vi "Eurotherm 32xx Series Temperature Control Monitoring.vi"() -> ()   [LabVIEW 2010]
doc: "This example demonstrates temperature control and monitoring.\n\nNote:\nBefore start this VI is it necessary:\n\n- preconfigure some specific parameters that are not supported by this driver (e.g. PV-I/O Type, Linearization type, Alarm Input Values... ) by Quick Codes, or by Eurotherm iTools or by instrument front panel controls\n- enter correct VISA Resource Descriptor, Device Address and Baud Rate into front-panel controls"
uses:
  <instrlib>/Eurotherm 32xx Series/Eurotherm 32xx Series.lvlib
panel:
  in  "Serial Configuration":T1={"Baud Rate (19200)"=19200, "Parity (0: None)"=0, "Break Length (0)"=20} {"Break Length (0)" items=["0"=10, "1.5"=15, "2.0"=20]; "Parity (0: None)" items=["None", "Odd", "Even"]; "Baud Rate (19200)" items=["1200"=1200, "2400"=2400, "4800"=4800, "9600"=9600, "19200"=19200]}
  in  "Alarm \nNumber (1)":u16=1 min=1 max=4
  out "Alarm Output":bool
  in  "Keylock":u8(ring) items=["None", "All", "Edit", "mod", "mAn", "Stby", "tmr"]
  in  "stop":bool
  out "Process Value - Chart":sgl(graph)
  out "Process Value":sgl
  in  "Setpoint Value":i16(slide) min=0 max=1300 scale=0.0..500.0
  in  "Controller  Mode":u8(ring) items=["Auto", "Manual"]
  in  "Unit Address (1)":u8=1 min=1 max=254
  in  "VISA resource name":refnum<visa-resource-name>
  in  "Acknowledge All Alarms":bool
  out "New ALARM !":bool
  # "(c) 2010 <Invensys Eurotherm>.  ALL RIGHTS RESERVED."
  # "Configuring Instrument\n \nPlease Wait......\n\nChart will update in 20 sec"
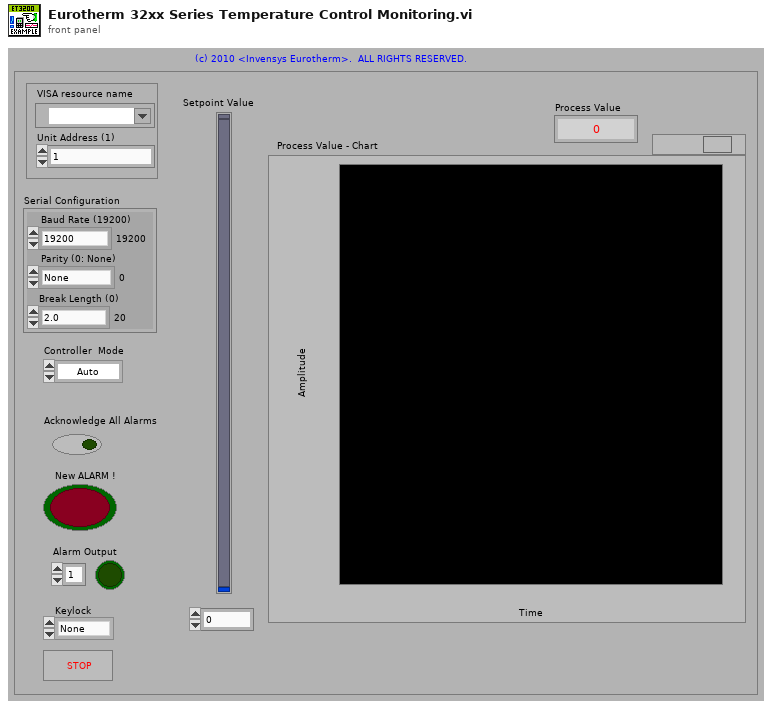
[diagram p1: front panel]
types:
  T1 = cluster{"Baud Rate (19200)":u32, "Parity (0: None)":u16, "Break Length (0)":u16}
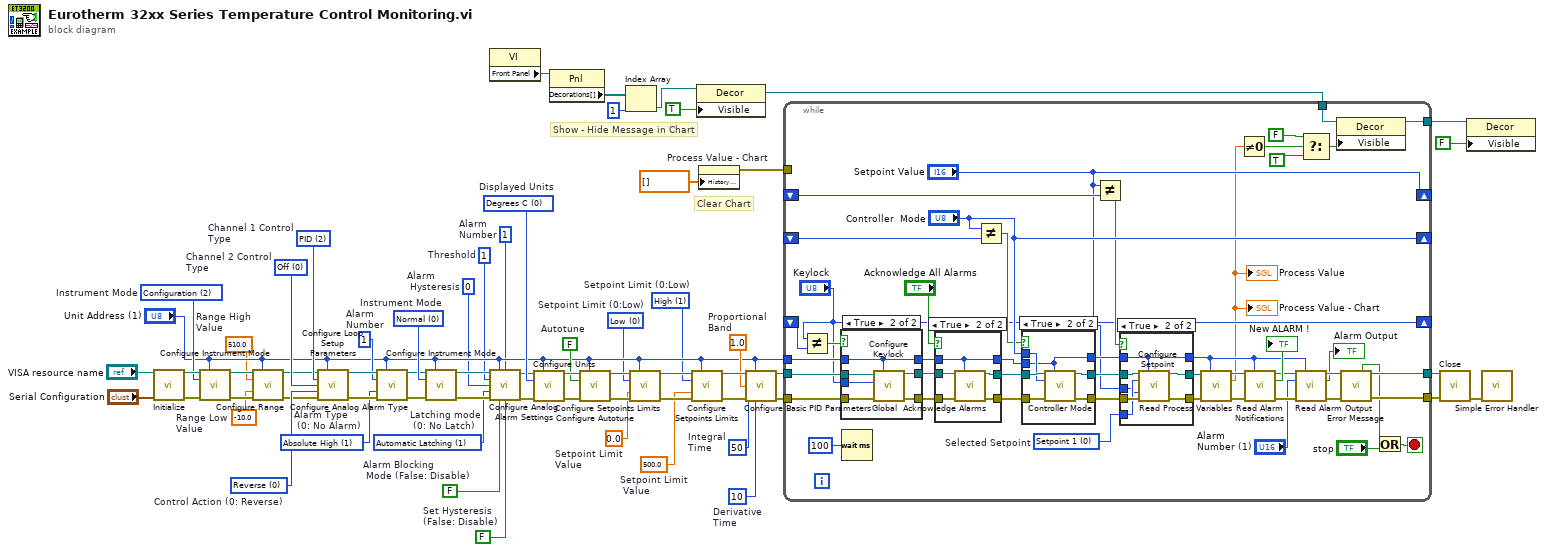
[diagram p0: block diagram]
diagram:
  w13 = sgl 500.0  # Setpoint Limit  Value
  w16 = sgl -10.0  # Range Low  Value
  w17 = sgl 510.0  # Range High Value
  w18 = u16 0 items=["Reverse", "Direct"]  # Control Action (0: Reverse)
  w19 = u16 0 items=["Low", "High"]  # Setpoint Limit (0:Low)
  w20 = u16 1 items=["Low", "High"]  # Setpoint Limit (0:Low)
  w23 = FALSE  # Set Hysteresis  (False: Disable)
  w34 = 10  # Derivative  Time
  w35 = 50  # Integral  Time
  w36 = sgl 1.0  # Proportional  Band
  w38 = sgl 0.0  # Setpoint Limit  Value
  w45 = FALSE  # Autotune
  w46 = u8 0 items=[" Degrees C", " Degrees F", " Degrees K"]  # Displayed Units
  w24 = FALSE  # Alarm Blocking  Mode (False: Disable)
  w26 = u16 1 items=["No Latch", "Automatic Latching", "Manual Latching", "Event Latching"]  # Latching mode  (0: No Latch)
  w27 = u16 0  # Alarm  Hysteresis
  w28 = u16 1  # Threshold
  w29 = u16 1  # Alarm  Number
  w51 = u8 1 items=["No Alarm", "Absolute High", "Absolute Low", "Deviation High", "Deviation Low", "Deviation Band", "Rising Rate of Change Alarm", "Falling Rate of Change Alarm"]  # Alarm Type  (0: No Alarm)
  w52 = u16 1  # Alarm  Number
  w57 = u8 0 items=["Normal", "StandBy", "Configuration"]  # Instrument Mode
  w58 = u8 0 items=["Off", "On/Off", "PID", "VPU", "VPB"]  # Channel 2 Control  Type
  w59 = u8 2 items=["Off", "On/Off", "PID", "VPU", "VPB"]  # Channel 1 Control  Type
  w62 = u8 2 items=["Normal", "StandBy", "Configuration"]  # Instrument Mode
  # "Show - Hide Message in Chart"
  # "Clear Chart"
  n1 = call <instrlib>:"Initialize.vi"("VISA resource name"="VISA resource name", "Serial Configuration"="Serial Configuration") -> ("VISA resource name out"=w63:refnum<visa-resource-name>, "error out"=w6:errorcluster)  [unwired: 12 in]
  n2 = call <instrlib>:"Configure Instrument Mode.vi"("VISA resource name"=w63, "Unit Address (1)"="Unit Address (1)", "Instrument Mode (0: Normal)"=w62, "error in (no error)"=w6) -> ("VISA resource name out"=w61:refnum<visa-resource-name>, "error out"=w60:errorcluster)  [unwired: 10 in]
  n3 = call <instrlib>:"Configure Range.vi"("VISA resource name"=w61, "Unit Address (1)"="Unit Address (1)", "Range High (0)"=w17, "Range Low (0)"=w16, "error in (no error)"=w60) -> ("VISA resource name out"=w15:refnum<visa-resource-name>, "error out"=w14:errorcluster)  [unwired: 9 in]
  n4 = call <instrlib>:"Configure Loop Setup Parameters.vi"("VISA resource name"=w15, "Unit Address (1)"="Unit Address (1)", "Channel 1 Control Algorithm (0: Off)"=w59, "Channel 2 Control Algorithm (0: Off)"=w58, "Control Action (0: Reverse)"=w18, "error in (no error)"=w14) -> ("VISA resource name out"=w56:refnum<visa-resource-name>, "error out"=w55:errorcluster)  [unwired: 8 in]
  n5 = call <instrlib>:"Configure Analog Alarm Type.vi"("VISA resource name"=w56, "Unit Address (1)"="Unit Address (1)", "Alarm Number (1)"=w52, "Alarm Type (0: No Alarm)"=w51, "error in (no error)"=w55) -> ("VISA resource name out"=w54:refnum<visa-resource-name>, "error out"=w53:errorcluster)  [unwired: 9 in]
  n6 = call <instrlib>:"Configure Instrument Mode.vi"("VISA resource name"=w54, "Unit Address (1)"="Unit Address (1)", "Instrument Mode (0: Normal)"=w57, "error in (no error)"=w53) -> ("VISA resource name out"=w32:refnum<visa-resource-name>, "error out"=w31:errorcluster)  [unwired: 10 in]
  n7 = property class="VI"() -> ("Front Panel"=w10:refnum<vi>)  [unwired: 2 in, 2 out]
  n8 = call <instrlib>:"Configure Analog Alarm Settings.vi"("VISA resource name"=w32, "Unit Address (1)"="Unit Address (1)", "Alarm Number (1)"=w29, "Threshold (0)"=w28, "Alarm Hysteresis (1)"=w27, "Latching Mode (0: No Latch)"=w26, "error in (no error)"=w31, "Enable Alarm Blocking (False: Disable)"=w24, "Enable Hysteresis (False: Disable)"=w23) -> ("VISA resource name out"=w22:refnum<visa-resource-name>, "error out"=w21:errorcluster)  [unwired: 5 in]
  n9 = call <instrlib>:"Configure Units.vi"("VISA resource name"=w22, "Unit Address (1)"="Unit Address (1)", "Displayed Units (0: Degrees C)"=w46, "error in (no error)"=w21) -> ("VISA resource name out"=w50:refnum<visa-resource-name>, "error out"=w49:errorcluster)  [unwired: 10 in]
  n10 = property class="Pnl"(reference=w10) -> ("Decorations[]"=w11:refnum<vi>[])  [unwired: 1 in, 2 out]
  n11 = call <instrlib>:"Configure Autotune.vi"("VISA resource name"=w50, "Unit Address (1)"="Unit Address (1)", "Enable Autotune  (False: Disable)"=w45, "error in (no error)"=w49) -> ("VISA resource name out"=w44:refnum<visa-resource-name>, "error out"=w43:errorcluster)  [unwired: 10 in]
  n12 = Index Array(array=w11, index=1) -> (element=w8:refnum<vi>)
  n13 = call <instrlib>:"Configure Setpoints Limits.vi"("VISA resource name"=w44, "Unit Address (1)"="Unit Address (1)", "Setpoint Limit (0:Low)"=w19, "Setpoint Limit Value (0)"=w38, "error in (no error)"=w43) -> ("VISA resource name out"=w48:refnum<visa-resource-name>, "error out"=w47:errorcluster)  [unwired: 9 in]
  n14 = call <instrlib>:"Configure Setpoints Limits.vi"("VISA resource name"=w48, "Unit Address (1)"="Unit Address (1)", "Setpoint Limit (0:Low)"=w20, "Setpoint Limit Value (0)"=w13, "error in (no error)"=w47) -> ("VISA resource name out"=w42:refnum<visa-resource-name>, "error out"=w39:errorcluster)  [unwired: 9 in]
  n15 = property class="Decor"(reference=w8, "Visible"=TRUE) -> (reference out=w7:refnum<vi>)  [unwired: 1 in, 1 out]
  n16 = property on="Process Value - Chart" class="WFChart (strict)"("History Data"=sgl[] []) -> (error out=w2:errorcluster)  [unwired: 2 in, 1 out]
  n17 = call <instrlib>:"Configure Basic PID Parameters.vi"("VISA resource name"=w42, "Unit Address (1)"="Unit Address (1)", "Proportional Band (1)"=w36, "Integral Time (1)"=w35, "error in (no error)"=w39, "Derivative Time (0)"=w34) -> ("VISA resource name out"=w41:refnum<visa-resource-name>, "error out"=w40:errorcluster)  [unwired: 8 in]
  n18 = while {
    tunnel: w41 -> [w83]
    tunnel: w40 -> [w82]
    tunnel: "Unit Address (1)" -> [w84]
    tunnel: [w104] -> w33
    tunnel: [w103] -> w37
    shift-right: ["Keylock"] -> _
    shift-left: _ -> [w93]
    shift-right: ["Controller  Mode"] -> _
    shift-left: _ -> [w90]
    shift-right: ["Setpoint Value"] -> _
    shift-left: _ -> [w88]
    tunnel: w7 -> [w68]
    tunnel: [w65] -> w4
    tunnel: w2 -> [_]
    stop <- w97 stop-if-true
    w99 = u8 0 items=["Setpoint 1", "Setpoint 2", "Alternate Setpoint", "Target Setpoint"]  # Selected Setpoint
    n19 = Not Equal?(x="Keylock", y=w93) -> (x != y?=w92:bool)
    n20 = case shown="True" w92 {
      tunnel: w83 -> [w141 w148]
      tunnel: w82 -> [w140 w147]
      tunnel: [w141 w146] -> w112
      tunnel: [w140 w145] -> w111
      tunnel: w84 -> [w142 w144]
      tunnel: [w142 w144] -> w101
      tunnel: "Keylock" -> [_ w143]
      frame False {
      }
      frame True {
        n21 = call <instrlib>:"Configure Keylock.vi"("VISA resource name"=w148, "Unit Address (1)"=w144, "Keylock"=w143, "error in (no error)"=w147) -> ("VISA resource name out"=w146:refnum<visa-resource-name>, "error out"=w145:errorcluster)  [unwired: 10 in]
      }
    }
    n22 = Wait (ms)(milliseconds to wait=u32 100) -> ()  [unwired: 1 out]
    n23 = case shown="True" "Acknowledge All Alarms" {
      tunnel: w112 -> [w133 w139]
      tunnel: w111 -> [w132 w138]
      tunnel: [w133 w137] -> w106
      tunnel: [w132 w136] -> w105
      tunnel: w101 -> [w134 w135]
      tunnel: [w134 w135] -> w100
      frame False {
      }
      frame True {
        n24 = call <instrlib>:"Global  Acknowledge Alarms.vi"("VISA resource name"=w139, "Unit Address (1)"=w135, "error in (no error)"=w138) -> ("VISA resource name out"=w137:refnum<visa-resource-name>, "error out"=w136:errorcluster)  [unwired: 11 in]
      }
    }
    n25 = Not Equal?(x="Controller  Mode", y=w90) -> (x != y?=w89:bool)
    n26 = case shown="True" w89 {
      tunnel: [w123 w131] -> w110
      tunnel: [w124 w130] -> w107
      tunnel: w106 -> [w124 w129]
      tunnel: w105 -> [w123 w128]
      tunnel: w100 -> [w125 w126]
      tunnel: "Controller  Mode" -> [_ w127]
      tunnel: [w125 w126] -> w98
      frame False {
      }
      frame True {
        n27 = call <instrlib>:"Controller Mode.vi"("VISA resource name"=w129, "Unit Address (1)"=w126, "Controller Mode (0: Auto)"=w127, "error in (no error)"=w128) -> ("VISA resource name out"=w130:refnum<visa-resource-name>, "error out"=w131:errorcluster)  [unwired: 10 in]
      }
    }
    n28 = Not Equal?(x="Setpoint Value", y=w88) -> (x != y?=w86:bool)
    n29 = case shown="True" w86 {
      tunnel: w110 -> [w113 w122]
      tunnel: [w113 w121] -> w109
      tunnel: [w114 w120] -> w108
      tunnel: w107 -> [w114 w119]
      tunnel: w99 -> [_ w118]
      tunnel: w98 -> [w115 w117]
      tunnel: [w115 w117] -> w73
      tunnel: "Setpoint Value" -> [_ w116]
      frame False {
      }
      frame True {
        n30 = call <instrlib>:"Configure Setpoint.vi"("VISA resource name"=w119, "Unit Address (1)"=w117, "Setpoint (0: Setpoint 1)"=w118, "Setpoint Value (0)"=w116, "error in (no error)"=w122) -> ("VISA resource name out"=w120:refnum<visa-resource-name>, "error out"=w121:errorcluster)  [unwired: 9 in]
      }
    }
    n31 = call <instrlib>:"Read Process Variables.vi"("VISA resource name"=w108, "Unit Address (1)"=w73, "error in (no error)"=w109) -> ("VISA resource name out"=w81:refnum<visa-resource-name>, "Process Value"=w66:sgl, "error out"=w80:errorcluster)  [unwired: 9 in, 1 out]
    "Process Value" <- w66
    "Process Value - Chart" <- w66
    n32 = Not Equal To 0?(x=w66) -> (x != 0?=w69:bool)
    n33 = call <instrlib>:"Read Alarm Notifications.vi"("VISA resource name"=w81, "Unit Address (1)"=w73, "error in (no error)"=w80) -> ("VISA resource name out"=w77:refnum<visa-resource-name>, "New Alarm"=→"New ALARM !":bool, "error out"=w78:errorcluster)  [unwired: 10 in]
    n34 = call <instrlib>:"Read Alarm Output.vi"("VISA resource name"=w77, "Unit Address (1)"=w73, "Alarm Number (1)"="Alarm \nNumber (1)", "error in (no error)"=w78) -> ("VISA resource name out"=w76:refnum<visa-resource-name>, "Alarm Output"=→"Alarm Output":bool, "error out"=w75:errorcluster)  [unwired: 9 in]
    n35 = Select(t=FALSE ("Visible"), s=w69, f=TRUE ("Visible")) -> (s? t:f=w71:bool)
    n36 = property class="Decor"(reference=w68, "Visible"=w71) -> (reference out=w65:refnum<vi>)  [unwired: 1 in, 1 out]
    n37 = call <instrlib>:"Error Message.vi"("VISA resource name"=w76, "error in (no error)"=w75) -> ("Status"=w95:bool, "VISA resource name out"=w104:refnum<visa-resource-name>, "error out"=w103:errorcluster)  [unwired: 9 in, 2 out]
    n38 = Or(x=w95, y="stop") -> (x .or. y?=w97:bool)
  }
  n39 = call <instrlib>:"Close.vi"("VISA resource name"=w33, "error in (no error)"=w37) -> ("error out"=w25:errorcluster)  [unwired: 13 in]
  n40 = property class="Decor"(reference=w4, "Visible"=FALSE) -> ()  [unwired: 1 in, 2 out]
  n41 = call <vilib>:"Simple Error Handler.vi"("error in (no error)"=w25) -> ()  [unwired: 4 in, 5 out]
